vi "get.vi"(7 "LabVIEW Web Service Request":refnum<class "Web Request.lvclass">) -> ()   [LabVIEW 2020]
uses:
  <vilib>/wsapi/Web Request.lvclass
panel:
  # "Use the Web Service Request input terminal to call the VIs on the Web Services palette. Do not remove it from the connector pane unless you don't need access to the palette."
  # "Each additional control wired to the connector pane will be available as an input in the URL. To include an indicator in terminal-mode output (the default setting), it must also be wired to the connector pane."
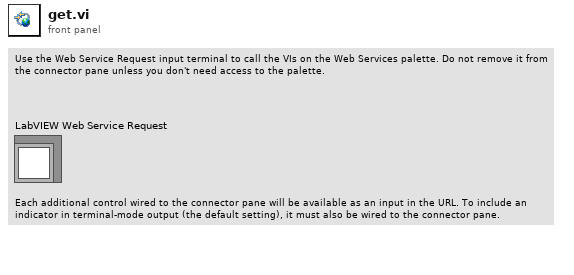
[diagram p1: front panel]
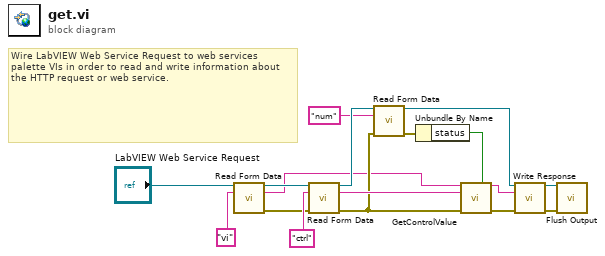
[diagram p0: block diagram]
diagram:
  # "Wire LabVIEW Web Service Request to web services palette VIs in order to read and write information about the HTTP request or web service."
  n1 = call <vilib>:"Read Form Data.vi"("LabVIEW Web Service Request"="LabVIEW Web Service Request", "key"="vi") -> ("LabVIEW Web Service Request out"=w14:refnum<class "Web Request.lvclass">, "value"=w1:string, "error out"=w7:errorcluster)  [unwired: 10 in, 1 out]
  n2 = call <vilib>:"Read Form Data.vi"("LabVIEW Web Service Request"=w14, "key"="ctrl", "error in (no error)"=w7) -> ("LabVIEW Web Service Request out"=w11:refnum<class "Web Request.lvclass">, "value"=w6:string, "error out"=w5:errorcluster)  [unwired: 9 in, 1 out]
  n3 = call <vilib>:"Read Form Data.vi"("LabVIEW Web Service Request"=w11, "key"="num", "error in (no error)"=w5) -> ("LabVIEW Web Service Request out"=w10:refnum<class "Web Request.lvclass">, "error out"=w8:errorcluster)  [unwired: 9 in, 2 out]
  n4 = Unbundle By Name(w8) -> ("status"=w4:bool)
  n5 = call "GetControlValue.vi"("vi"=w1, "UseEnum (true)"=w4, "ctrl"=w6, "error in (no error)"=w5) -> ("String out"=w2:string, "error out"=w3:errorcluster)  [unwired: 9 in, 1 out]
  n6 = call <vilib>:"Write Response.vi"("LabVIEW Web Service Request"=w10, "response string"=w2, "error in (no error)"=w3) -> ("LabVIEW Web Service Request out"=w13:refnum<class "Web Request.lvclass">, "error out"=w12:errorcluster)  [unwired: 11 in]
  n7 = call <vilib>:"Flush Output.vi"("LabVIEW Web Service Request"=w13, "error in (no error)"=w12) -> ()  [unwired: 12 in, 2 out]
